vi "Edit Tolerance Limits (Part Selection Distinguished).vi"(8 "error in (no error)":errorcluster, 11 "ZenGage v3.0 UI in":refnum<class "ZenGage v3.0 UI.lvclass">) -> (0 "error out":errorcluster, 2 "Parts List out":string[](array[string]), 3 "ZenGage v3.0 UI out":refnum<class "ZenGage v3.0 UI.lvclass">)   [LabVIEW 2015, in "ZenGage v3.0 UI.lvclass"]
uses:
  ZenGage v3.0 UI.lvclass
  ZenGage v3.0 UI.lvclass/ZenGage v3.0 UI.ctl
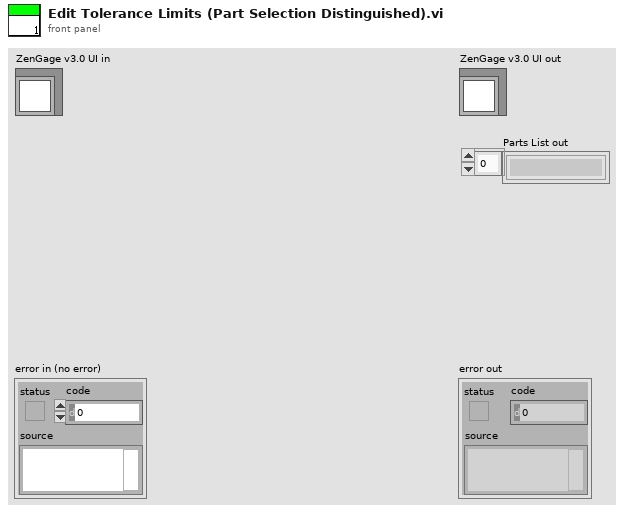
[diagram p1: front panel]
types:
  T1 = enum32{"Analytics", "Blank", "Diagnostics", "Run", "Edit Tolerance Settings"}
  T2 = enum8{"Enabled", "Disabled", "Disabled and Grayed Out"}
  T3 = cluster{"Part Name":string, "Operator Number":string, "Order Number":string}
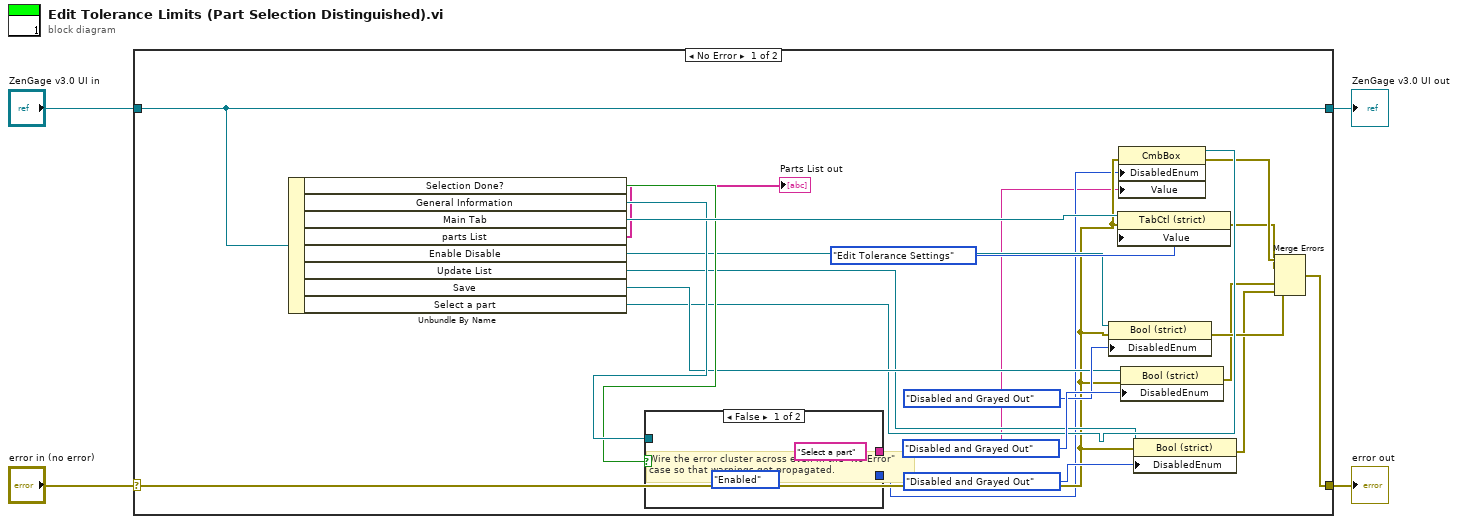
[diagram p0: block diagram]
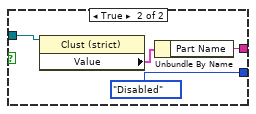
[diagram p2: hidden frame]
diagram:
  n1 = case shown="No Error" "error in (no error)" {
    selector: "error in (no error)" -> [w13 w34]
    tunnel: [w5 w34] -> w3
    tunnel: [w26 w33] -> w1
    tunnel: "ZenGage v3.0 UI in" -> [w26 w33]
    frame No Error {
      # "Wire the error cluster across even in the \"No Error\"\ncase so that warnings get propagated."
      n2 = Unbundle By Name(w26) -> ("Selection Done?"=w19:bool, "General Information"=w20:refnum<vi>, "Main Tab"=w22:refnum<vi>, "parts List"=→"Parts List out":string[], "Enable Disable"=w15:refnum<vi>, "Update List"=w16:refnum<vi>, "Save"=w18:refnum<vi>, "Select a part"=w17:refnum<vi>)
      n3 = case shown="False" w19 {
        tunnel: [T2."Enabled" ("Disabled") T2."Disabled" ("Disabled")] -> w12
        tunnel: w20 -> [_ w31]
        tunnel: ["Select a part" ("Part Name") w29] -> w11
        frame False {
        }
        frame True {
          n4 = property class="Clust (strict)"(reference=w31) -> ("Value"=w30:T3)  [unwired: 1 in, 2 out]
          n5 = Unbundle By Name(w30) -> ("Part Name"=w29:string)
        }
      }
      n6 = property class="Bool (strict)"(reference=w15, error in=w13, "DisabledEnum"=T2."Disabled and Grayed Out" ("Disabled")) -> (error out=w8:errorcluster)  [unwired: 1 out]
      n7 = property class="TabCtl (strict)"(reference=w22, error in=w13, "Value"=T1."Edit Tolerance Settings") -> (error out=w9:errorcluster)  [unwired: 1 out]
      n8 = property class="CmbBox"(reference=w17, error in=w13, "DisabledEnum"=w12, "Value"=w11) -> (error out=w10:errorcluster)  [unwired: 1 out]
      n9 = property class="Bool (strict)"(reference=w18, error in=w13, "DisabledEnum"=T2."Disabled and Grayed Out" ("Disabled")) -> (error out=w7:errorcluster)  [unwired: 1 out]
      n10 = property class="Bool (strict)"(reference=w16, error in=w13, "DisabledEnum"=T2."Disabled and Grayed Out" ("Disabled")) -> (error out=w6:errorcluster)  [unwired: 1 out]
      n11 = Merge Errors(w10, w9, w8, w7, w6) -> (w5:errorcluster)
    }
    frame Error {
    }
  }
  "error out" <- w3
  "ZenGage v3.0 UI out" <- w1
